vi "X middle row transform.vi"(10 "Pretransform Rubix Array":T1[][](array[typedef]), 11 "Command":T2=-1 items=["Up"=-1, "Down"=1]) -> (1 "Axis":cluster{"X":sgl, "Y":sgl, "Z":sgl}={"X"=1.0, "Y"=0.0, "Z"=0.0}, 2 "Transform Rubix Array":T1[][](array[typedef]), 3 "Facets to move":T1[](array[typedef]))   [LabVIEW 2019]
uses:
  Rotate array command.ctl
  Rubix Array data type.ctl
  section movement.ctl
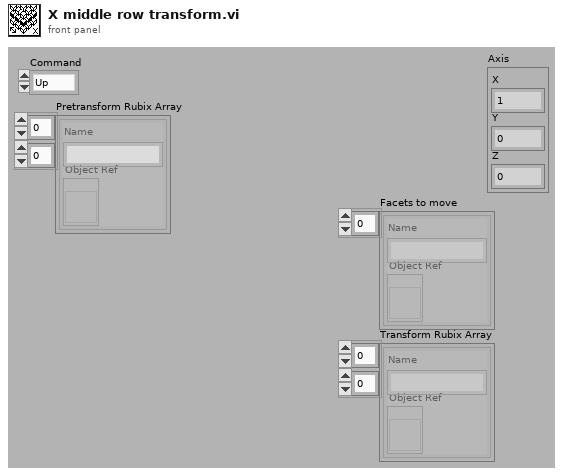
[diagram p1: front panel]
types:
  T1 = typedef "Rubix Array data type.ctl" = cluster{"Object Ref":refnum<vi>, "Name":string}
  T2 = typedef "Rotate array command.ctl" = i32
  T3 = typedef "section movement.ctl" = enum16{"Left", "Right"}
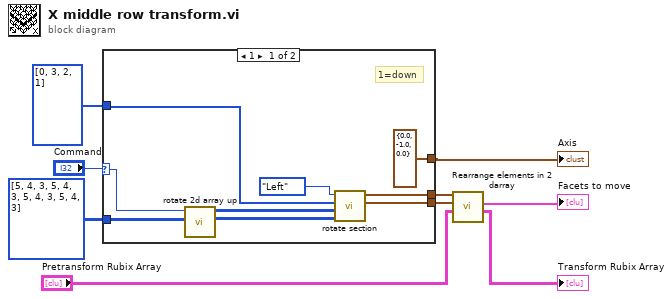
[diagram p0: block diagram]
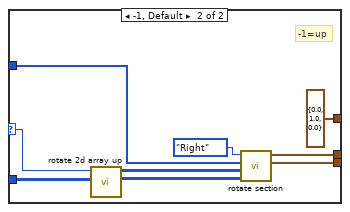
[diagram p2: hidden frame]
diagram:
  n1 = case shown="1" "Command" {
    selector: "Command" -> [w10 w19]
    tunnel: [w17 w26] -> w9
    tunnel: [w16 w25] -> w8
    tunnel: i32[][] [[5, 4, 3], [5, 4, 3], [5, 4, 3], [5, 4, 3]] ("From Facet") -> [w14 w23]
    tunnel: i32[] [0, 3, 2, 1] ("From 2") -> [w11 w21]
    tunnel: [cluster{"X":sgl, "Y":sgl, "Z":sgl} {"X"=0.0, "Y"=-1.0, "Z"=0.0} ("Axis") cluster{"X":sgl, "Y":sgl, "Z":sgl} {"X"=0.0, "Y"=1.0, "Z"=0.0} ("Axis")] -> w3
    frame 1 {
      # "1=down"
      n2 = call "rotate 2d array up.vi"("From Facet"=w14, "Ring"=w10) -> ("Rotated"=w15:i32[][], "Dup Original"=w13:i32[][])  [unwired: 8 in]
      n3 = call "rotate section.vi"("To Facet"=w15, "From Facet"=w13, "From"=w11, "Enum"=section_movement."Left") -> ("To"=w16:cluster{"row":i32, "column":i32}[], "From"=w17:cluster{"row":i32, "column":i32}[])  [unwired: 6 in]
    }
    frame -1, Default {
      # "-1=up"
      n4 = call "rotate 2d array up.vi"("From Facet"=w23, "Ring"=w19) -> ("Rotated"=w24:i32[][], "Dup Original"=w22:i32[][])  [unwired: 8 in]
      n5 = call "rotate section.vi"("To Facet"=w24, "From Facet"=w22, "From"=w21, "Enum"=section_movement."Right") -> ("To"=w25:cluster{"row":i32, "column":i32}[], "From"=w26:cluster{"row":i32, "column":i32}[])  [unwired: 6 in]
    }
  }
  "Axis" <- w3
  n6 = call "Rearrange elements in 2 darray.vi"("Pretransform Rubix Array"="Pretransform Rubix Array", "To"=w8, "From"=w9) -> ("Transform Rubix Array"=→"Transform Rubix Array":T1[][], "Facets to move"=→"Facets to move":T1[])  [unwired: 7 in]
